vi "Syntax Check & RPN.vi"(8 "error in (no error)":errorcluster, 11 "STEP in":T1) -> (0 "error out":errorcluster, 3 "STEP out":T1)   [LabVIEW 2014, in "SeqLoop.lvlib"]
uses:
  TypeDefs/STEP.ctl
  TypeDefs/LogicParsedExpression.ctl
  Mimico Display/TypeDefs/Mimic Data.ctl
  Mimico Display/TypeDefs/BG Image.ctl
  Mimico Display/TypeDefs/mObject.ctl
  SeqLoop.lvlib
  Mimico Display/Mimico Display.lvlib
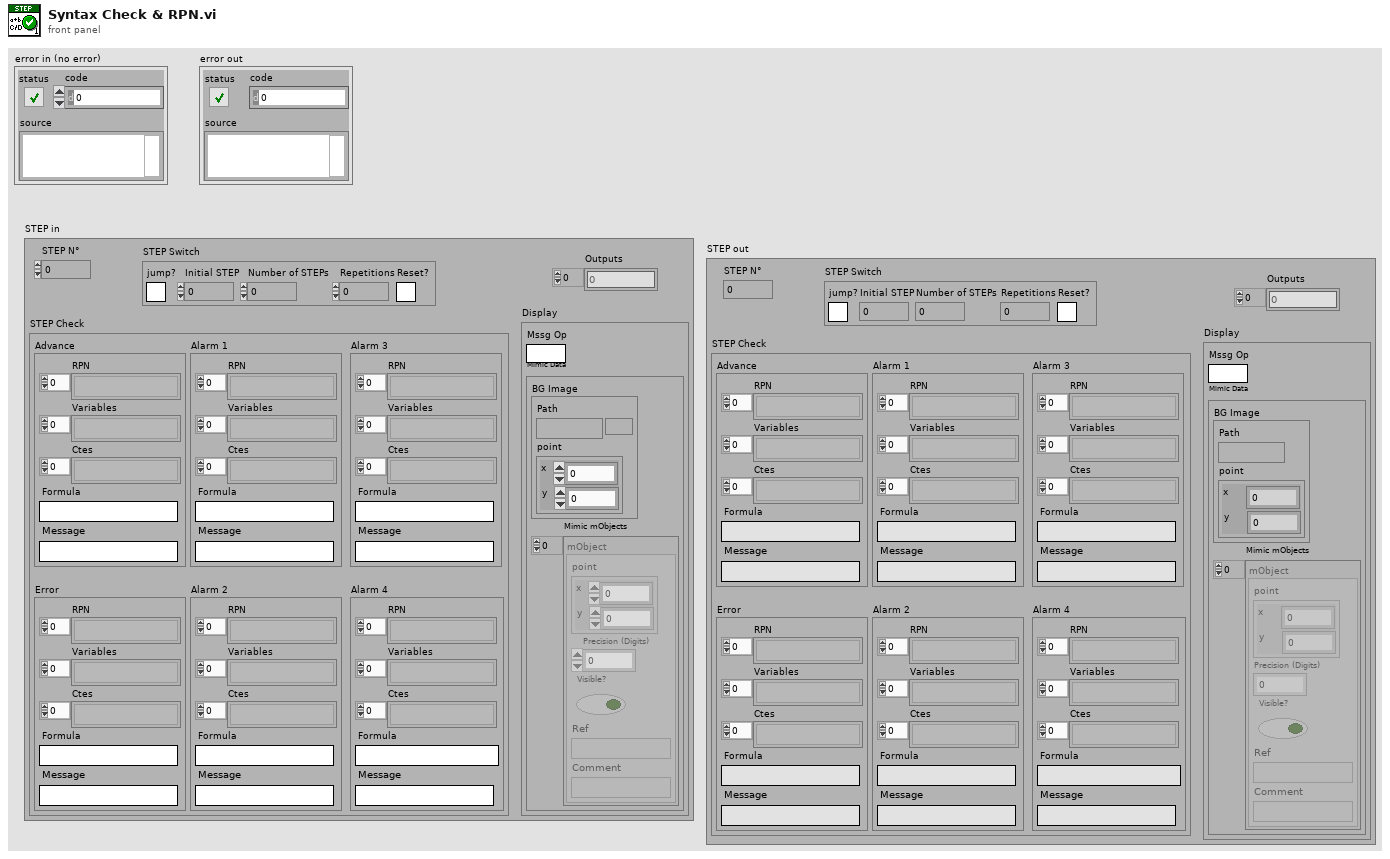
[diagram p1: front panel]
types:
  T1 = typedef "SeqLoop.lvlib/STEP.ctl" = cluster{"STEP N°":u32, "STEP Switch":cluster{"jump?":bool, "Initial STEP":u32, "Number of STEPs":u32, "Repetitions":u32, "Reset?":bool}, "Outputs":i32[], "STEP Check":cluster{"Advance":T2, "Error ":T2, "Alarm 1":T2, "Alarm 2":T2, "Alarm 3":T2, "Alarm 4":T2}, "Display":cluster{"Mssg Op":string, "Mimic Data":T3}}
  T2 = typedef "SeqLoop.lvlib/LogicParsedExpression.ctl" = cluster{"RPN ":string[], "Variables":string[], "Ctes":string[], "Formula":string, "Message":string}
  T3 = typedef "SeqLoop.lvlib/Mimico Display.lvlib/Mimic Data.ctl" = cluster{"BG Image":T4, "Mimic mObjects":T5[]}
  T4 = typedef "SeqLoop.lvlib/Mimico Display.lvlib/BG Image.ctl" = cluster{"Path":path, "point":cluster{"x":i16, "y":i16}}
  T5 = typedef "SeqLoop.lvlib/Mimico Display.lvlib/mObject.ctl" = cluster{"point":cluster{"x":i16, "y":i16}, "Precision (Digits)":i32, "Visible?":bool, "Ref":string, "Comment":string}
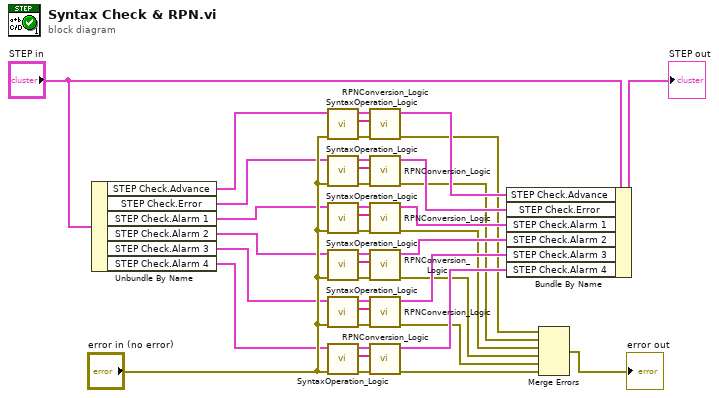
[diagram p0: block diagram]
diagram:
  n1 = Unbundle By Name("STEP in") -> ("STEP Check.Advance"=w4:T2, "STEP Check.Error"=w5:T2, "STEP Check.Alarm 1"=w6:T2, "STEP Check.Alarm 2"=w7:T2, "STEP Check.Alarm 3"=w8:T2, "STEP Check.Alarm 4"=w9:T2)
  n2 = call "SyntaxOperation_Logic.vi"("error in (no error)"="error in (no error)", "Logical Parsed Expression"=w4) -> ("error out"=w11:errorcluster, "Token"=w10:string[], "Logical Parsed Expression Out"=w3:T2)  [unwired: 6 in, 1 out]
  n3 = call "SyntaxOperation_Logic.vi"("error in (no error)"="error in (no error)", "Logical Parsed Expression"=w5) -> ("error out"=w14:errorcluster, "Token"=w13:string[], "Logical Parsed Expression Out"=w12:T2)  [unwired: 6 in, 1 out]
  n4 = call "SyntaxOperation_Logic.vi"("error in (no error)"="error in (no error)", "Logical Parsed Expression"=w6) -> ("error out"=w15:errorcluster, "Token"=w17:string[], "Logical Parsed Expression Out"=w16:T2)  [unwired: 6 in, 1 out]
  n5 = call "SyntaxOperation_Logic.vi"("error in (no error)"="error in (no error)", "Logical Parsed Expression"=w7) -> ("error out"=w20:errorcluster, "Token"=w19:string[], "Logical Parsed Expression Out"=w18:T2)  [unwired: 6 in, 1 out]
  n6 = call "SyntaxOperation_Logic.vi"("error in (no error)"="error in (no error)", "Logical Parsed Expression"=w8) -> ("error out"=w23:errorcluster, "Token"=w22:string[], "Logical Parsed Expression Out"=w21:T2)  [unwired: 6 in, 1 out]
  n7 = call "SyntaxOperation_Logic.vi"("error in (no error)"="error in (no error)", "Logical Parsed Expression"=w9) -> ("error out"=w26:errorcluster, "Token"=w25:string[], "Logical Parsed Expression Out"=w24:T2)  [unwired: 6 in, 1 out]
  n8 = call "RPNConversion_Logic.vi"("error in"=w11, "Token"=w10, "Logical Parsed Expression"=w3) -> ("error out"=w33:errorcluster, "Logical Parsed Expression Out"=w35:T2)  [unwired: 7 in]
  n9 = call "RPNConversion_Logic.vi"("error in"=w14, "Token"=w13, "Logical Parsed Expression"=w12) -> ("error out"=w32:errorcluster, "Logical Parsed Expression Out"=w36:T2)  [unwired: 7 in]
  n10 = call "RPNConversion_Logic.vi"("error in"=w15, "Token"=w17, "Logical Parsed Expression"=w16) -> ("error out"=w31:errorcluster, "Logical Parsed Expression Out"=w37:T2)  [unwired: 7 in]
  n11 = call "RPNConversion_Logic.vi"("error in"=w20, "Token"=w19, "Logical Parsed Expression"=w18) -> ("error out"=w30:errorcluster, "Logical Parsed Expression Out"=w38:T2)  [unwired: 7 in]
  n12 = call "RPNConversion_Logic.vi"("error in"=w23, "Token"=w22, "Logical Parsed Expression"=w21) -> ("error out"=w29:errorcluster, "Logical Parsed Expression Out"=w39:T2)  [unwired: 7 in]
  n13 = call "RPNConversion_Logic.vi"("error in"=w26, "Token"=w25, "Logical Parsed Expression"=w24) -> ("error out"=w28:errorcluster, "Logical Parsed Expression Out"=w40:T2)  [unwired: 7 in]
  n14 = Bundle By Name(cluster="STEP in", "STEP Check.Advance"=w35, "STEP Check.Error"=w36, "STEP Check.Alarm 1"=w37, "STEP Check.Alarm 2"=w38, "STEP Check.Alarm 3"=w39, "STEP Check.Alarm 4"=w40) -> (→"STEP out":T1)
  n15 = Merge Errors(w33, w32, w31, w30, w29, w28) -> (→"error out":errorcluster)
